vi "rs3_decimate_color.vi"(7 "Decimate":u8=3 min=1 max=30, 8 "Input X":i32=1280, 9 "Input Y":i32=720, 10 "Color format":enum16{"Monochrome", "RGB internal (RGB)"}(ring)=enum."RGB internal (RGB)", 11 "input image":u8[](array[numeric])=array[2764800 elements]) -> (0 "NewX":i32, 1 "NewY":i32, 3 "decimated color":u8[](array[numeric]))   [LabVIEW 2017, in "libRealSense3.lvlib"]
doc: "Subsamples the color (monochrome or RGB) by a decimation factor.\nIt pads to make x, y multiples of 2."
uses:
  libRealSense3.lvlib
panel:
  out "zero pad":bool
  in  "error in (no error)":errorcluster
  out "error out":errorcluster
  # "RS3_Decimate Color"
  # "Multiple of 2"
  # "(C) 2017 Intel Corp.,  AGJ"
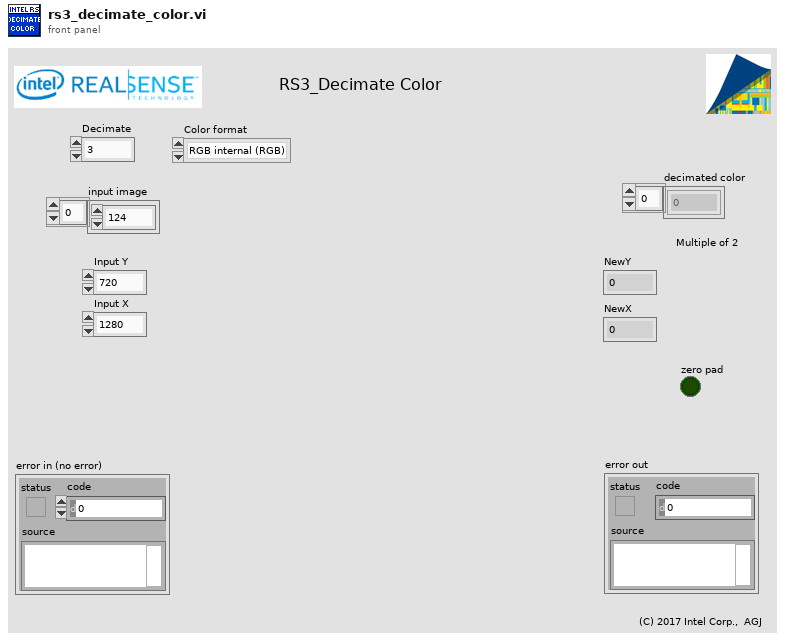
[diagram p1: front panel]
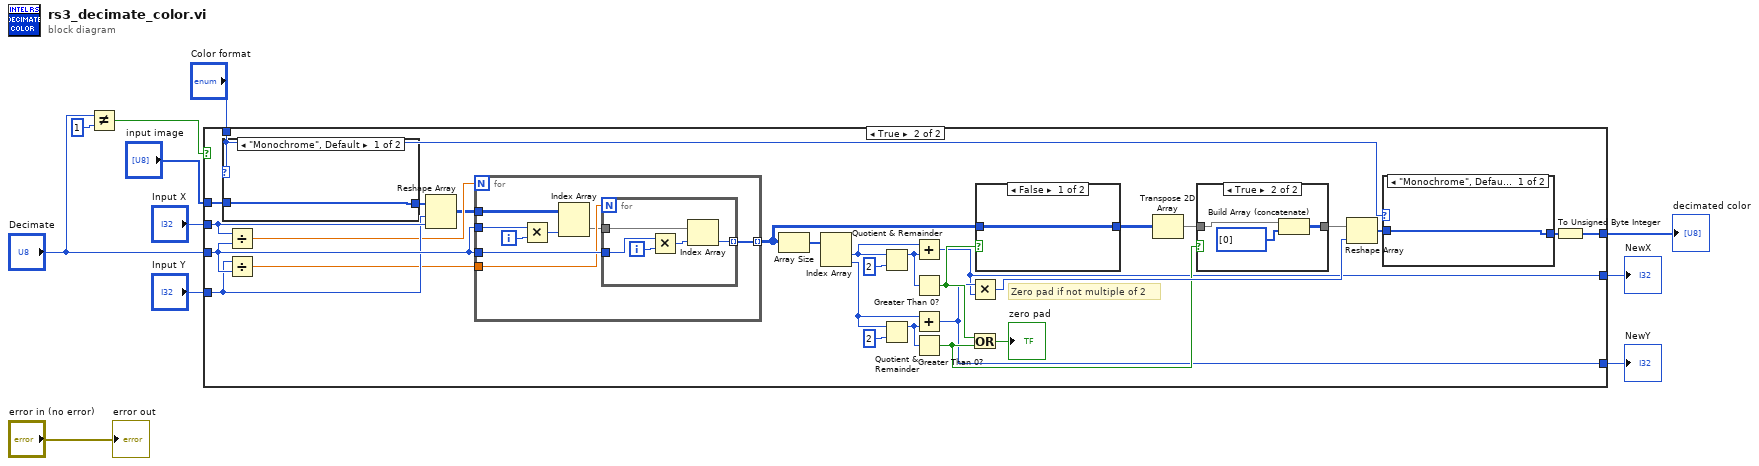
[diagram p0: block diagram]
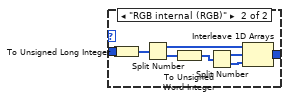
[diagram p3: hidden frame]
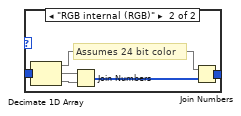
[diagram p4: hidden frame]
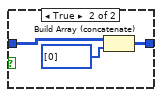
[diagram p6: hidden frame]
diagram:
  n1 = Not Equal?(x="Decimate", y=1) -> (x != y?=w4:bool)
  n2 = case shown="True" w4 {
    tunnel: "Decimate" -> [_ w39]
    tunnel: [w14 w38] -> w8
    tunnel: "Input X" -> [w13 w37]
    tunnel: "Input Y" -> [w12 w36]
    tunnel: "input image" -> [w14 w35]
    tunnel: [w13 w16] -> w3
    tunnel: [w12 w17] -> w2
    tunnel: "Color format" -> [_ w15]
    frame False {
    }
    frame True {
      # "Zero pad if not multiple of 2"
      n3 = case shown="\"Monochrome\", Default" w15 {
        tunnel: [w53 w55] -> w43
        tunnel: w35 -> [w53 w54]
        frame "Monochrome", Default {
        }
        frame "RGB internal (RGB)" {
          # "Assumes 24 bit color"
          n4 = Decimate 1D Array(w54) -> (w58:u8[], w57:u8[], w56:u8[])
          n5 = Join Numbers(hi=w57, lo=w56) -> ((hi.lo)=w59:u16[])
          n6 = Join Numbers(hi=w58, lo=w59) -> ((hi.lo)=w55:u32[])
        }
      }
      n7 = Divide(x=w37, y=w39) -> (x/y=w34:dbl)
      n8 = Divide(x=w36, y=w39) -> (x/y=w18:dbl)
      n9 = Reshape Array(w43, w36, w37) -> (w33:u32[][])
      n10 = for {
        N: w34 -> [_]
        tunnel: w39 -> [w74]
        tunnel: w39 -> [w73]
        tunnel: w18 -> [w72]
        tunnel: w33 -> [w71]
        tunnel: [w69] -> w23 mode=indexing
        i -> [w75]
        n11 = Multiply(x=w74, y=w75) -> (x*y=w68:i32)
        n12 = Index Array(array=w71, index (col)=w68) -> (element=w70:u32[])  [unwired: 1 in]
        n13 = for {
          N: w72 -> [_]
          tunnel: w73 -> [w79]
          tunnel: w70 -> [w78]
          tunnel: [w76] -> w69 mode=indexing
          i -> [w80]
          n14 = Multiply(x=w79, y=w80) -> (x*y=w77:i32)
          n15 = Index Array(array=w78, index=w77) -> (element=w76:u32)
        }
      }
      n16 = Array Size(array=w23) -> (size(s)=w28:i32[])
      n17 = Index Array(array=w28) -> (element #1=w32:i32, element #2=w31:i32)  [unwired: 2 in]
      n18 = Quotient & Remainder(x=w32, y=2) -> (x-y*floor(x/y)=w27:i32)  [unwired: 1 out]
      n19 = Quotient & Remainder(x=w31, y=2) -> (x-y*floor(x/y)=w26:i32)  [unwired: 1 out]
      n20 = Add(x=w32, y=w27) -> (x+y=w16:i32)
      n21 = Greater Than 0?(x=w27) -> (x > 0?=w24:bool)
      n22 = Add(x=w31, y=w26) -> (x+y=w17:i32)
      n23 = Greater Than 0?(x=w26) -> (x > 0?=w21:bool)
      n24 = Multiply(x=w17, y=w16) -> (x*y=w42:i32)
      n25 = Or(x=w24, y=w21) -> (x .or. y?=→"zero pad":bool)
      n26 = case shown="False" w24 {
        tunnel: w23 -> [w64 w66]
        tunnel: [w64 w65] -> w22
        frame False {
        }
        frame True {
          n27 = Build Array (concatenate)(w66, u32[] [0]) -> (w65:u32[][])
        }
      }
      n28 = Transpose 2D Array(2D array=w22) -> (transposed array=w20:u32[][])
      n29 = case shown="True" w21 {
        tunnel: w20 -> [w60 w62]
        tunnel: [w60 w61] -> w19
        frame False {
        }
        frame True {
          n30 = Build Array (concatenate)(w62, u32[] [0]) -> (w61:u32[][])
        }
      }
      n31 = Reshape Array(w19, w42) -> (w41:u32[])
      n32 = case shown="\"Monochrome\", Default" w15 {
        tunnel: w41 -> [w44 w46]
        tunnel: [w44 w45] -> w40
        frame "Monochrome", Default {
        }
        frame "RGB internal (RGB)" {
          n33 = To Unsigned Long Integer(number=w46) -> (unsigned 32bit integer=w52:u32[])
          n34 = Split Number(x=w52) -> (hi(x)=w49:u16[], lo(x)=w51:u16[])
          n35 = To Unsigned Word Integer(number=w51) -> (unsigned 16bit integer=w50:u16[])
          n36 = Split Number(x=w50) -> (hi(x)=w48:u8[], lo(x)=w47:u8[])
          n37 = Interleave 1D Arrays(w49, w48, w47) -> (w45:u16[])
        }
      }
      n38 = To Unsigned Byte Integer(number=w40) -> (unsigned 8bit integer=w38:u8[])
    }
  }
  "decimated color" <- w8
  "NewX" <- w3
  "NewY" <- w2
  "error out" <- "error in (no error)"
